vi "SubVI_Grab_Target_Level_Mode.vi"(8 "error in (no error)":errorcluster) -> (0 "error out":errorcluster, 1 "Target Array":dbl[](array[numeric]), 2 "Current level":dbl, 3 "Task":i32, 4 "HAND":string, 6 "MODE":string)   [LabVIEW 2020]
uses:
  Global 1.vi
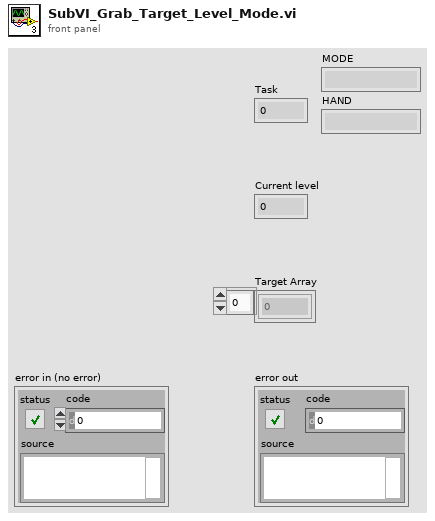
[diagram p1: front panel]
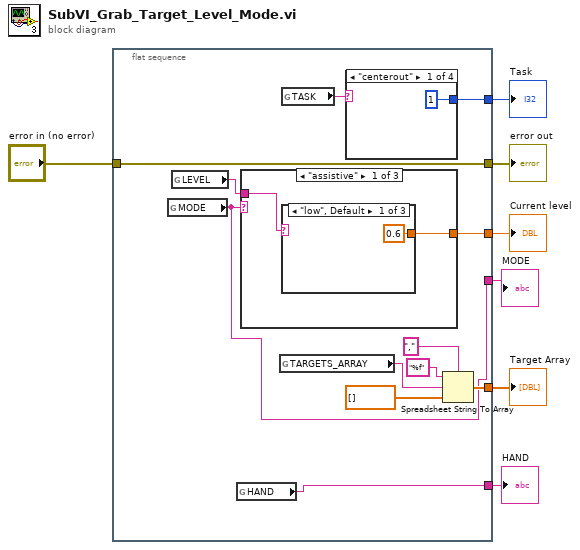
[diagram p0: block diagram]
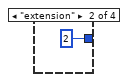
[diagram p2: hidden frame]
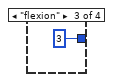
[diagram p3: hidden frame]
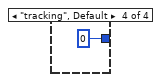
[diagram p4: hidden frame]
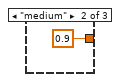
[diagram p5: hidden frame]
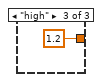
[diagram p6: hidden frame]
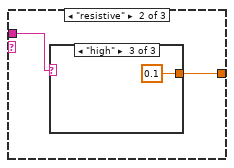
[diagram p7: hidden frame]
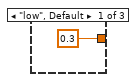
[diagram p8: hidden frame]
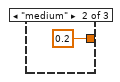
[diagram p9: hidden frame]
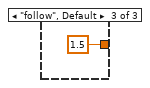
[diagram p10: hidden frame]
diagram:
  n1 = flat-sequence {
    tunnel: [w15] -> w4
    tunnel: [w13] -> w5
    tunnel: [w12] -> w3
    tunnel: "error in (no error)" -> [w10]
    tunnel: [w10] -> w7
    tunnel: [w9] -> w2
    tunnel: [w8] -> w1
    frame #0 {
      n2 = global read "Global 1.vi" "MODE"() -> (w9:string)
      n3 = global read "Global 1.vi" "LEVEL"() -> (w14:string)
      n4 = global read "Global 1.vi" "HAND"() -> (w8:string)
      n5 = case shown="\"assistive\"" w9 {
        tunnel: [w25 w30 1.5] -> w13
        tunnel: w14 -> [w24 w29 _]
        frame "assistive" {
          n6 = case shown="\"low\", Default" w24 {
            tunnel: [0.6 0.9 1.2] -> w25
            frame "low", Default {
            }
            frame "medium" {
            }
            frame "high" {
            }
          }
        }
        frame "resistive" {
          n7 = case shown="\"high\"" w29 {
            tunnel: [0.3 0.2 0.1] -> w30
            frame "low", Default {
            }
            frame "medium" {
            }
            frame "high" {
            }
          }
        }
        frame "follow", Default {
        }
      }
      n8 = global read "Global 1.vi" "TARGETS_ARRAY"() -> (w19:string)
      n9 = global read "Global 1.vi" "TASK"() -> (w11:string)
      n10 = case shown="\"centerout\"" w11 {
        tunnel: [1 2 3 0] -> w12
        frame "centerout" {
        }
        frame "extension" {
        }
        frame "flexion" {
        }
        frame "tracking", Default {
        }
      }
      n11 = Spreadsheet String To Array(delimiter (Tab)=",", format string="%f", spreadsheet string=w19, array type (2D Dbl)=dbl[] []) -> (array=w15:dbl[])
    }
  }
  "error out" <- w7
  "Current level" <- w5
  "Target Array" <- w4
  "Task" <- w3
  "MODE" <- w2
  "HAND" <- w1
